vi "WritingAttributes.vi"(0 "reference in":refnum<class "MyG#SubClass.lvclass">, 2 "increment":dbl, 5 "error in (no error)":errorcluster) -> (14 "reference out":refnum<class "MyG#SubClass.lvclass">, 19 "error out":errorcluster)   [LabVIEW 2020, in "MyG#SubClass.lvclass"]
uses:
  MyG#SubClass.lvclass
  C:/Program Files (x86)/National Instruments/LabVIEW 2020/examples/AddQ/G#/CreateDestroy/MyG#Class_class/MyG#Class.lvclass
  MyG#Class_class/MyG#Class.lvclass
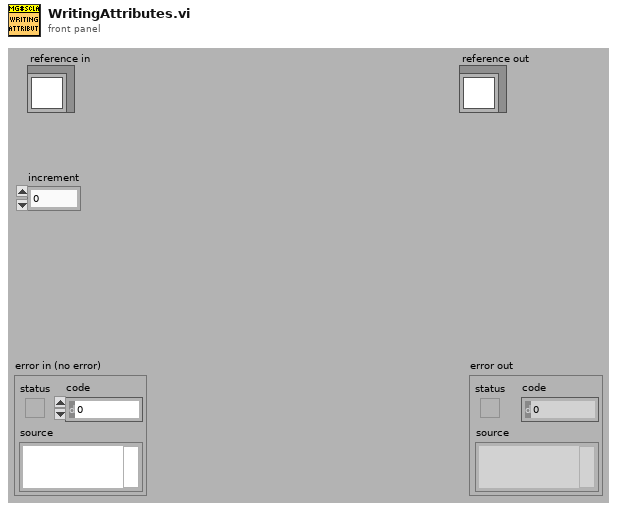
[diagram p1: front panel]
types:
  T1 = typedef "MyG#Class.lvclass/ObjectAttributesRef.ctl" = refnum<data-value>
  T2 = typedef "MyG#SubClass.lvclass/ObjectAttributesRef.ctl" = refnum<data-value>
  T3 = typedef "MyG#SubClass.lvclass/ObjectAttributes.ctl" = cluster{"MySubAttribute":dbl}
  T4 = typedef "MyG#Class.lvclass/ObjectAttributes.ctl" = cluster{"MyAttribute":dbl}
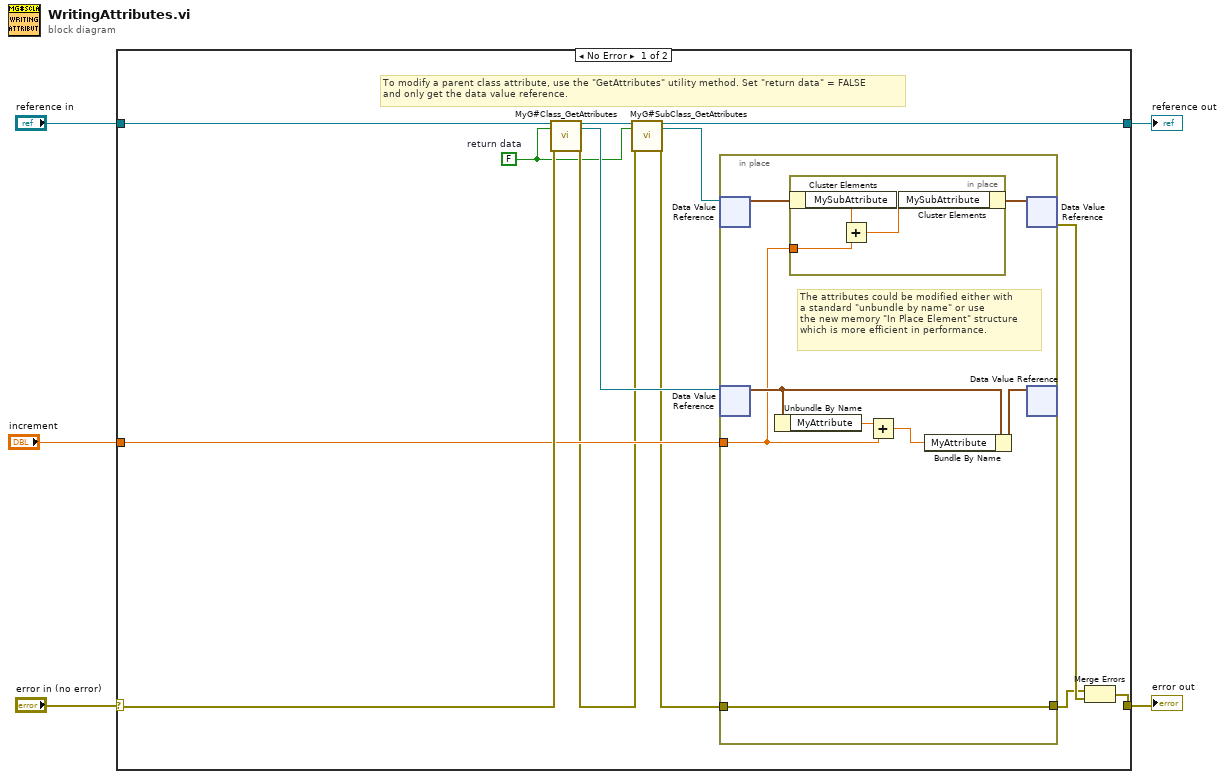
[diagram p0: block diagram]
diagram:
  n1 = case shown="No Error" "error in (no error)" {
    selector: "error in (no error)" -> [w14 w31]
    tunnel: [w18 w31] -> w4
    tunnel: [w8 w30] -> w2
    tunnel: "reference in" -> [w15 w30]
    tunnel: "increment" -> [w12 _]
    frame No Error {
      w7 = FALSE  # return data
      # "To modify a parent class attribute, use the \"GetAttributes\" utility method. Set \"return data\" = FALSE\nand only get the data value reference."
      n2 = call "MyG#Class_GetAttributes.vi"("reference in"=w15, "return data? (T)"=w7, "error in (no error)"=w14) -> ("reference out"=w11:refnum<class "MyG#SubClass.lvclass">, "attributes ref"=w13:T1, "error out"=w10:errorcluster)  [unwired: 13 in, 1 out]
      n3 = call "MyG#SubClass_GetAttributes.vi"("reference in"=w11, "return data? (T)"=w7, "error in (no error)"=w10) -> ("reference out"=w8:refnum<class "MyG#SubClass.lvclass">, "attributes ref"=w6:T2, "error out"=w9:errorcluster)  [unwired: 13 in, 1 out]
      n4 = in-place {
        in-place-border: w9 -> [w24]
        in-place-border: [w24] -> w16
        in-place-border: w12 -> [w19]
        # "The attributes could be modified either with\na standard \"unbundle by name\" or use\nthe new memory \"In Place Element\" structure\nwhich is more efficient in performance."
        n5 = in-place-dvr #1(w6) -> (w25:T3)  [unwired: 1 out]
        n6 = in-place-dvr #2(w13) -> (w22:T4)  [unwired: 1 out]
        n7 = Unbundle By Name(w22) -> ("MyAttribute"=w21:dbl)
        n8 = in-place {
          in-place-border: w19 -> [w28]
          n9 = in-place-cluster #3(w25) -> ("MySubAttribute"=w29:dbl)
          n10 = Add(x=w29, y=w28) -> (x+y=w27:dbl)
          n11 = in-place-cluster #3("MySubAttribute"=w27) -> (w26:T3)
        }
        n12 = Add(x=w21, y=w19) -> (x+y=w20:dbl)
        n13 = Bundle By Name(cluster=w22, "MyAttribute"=w20) -> (w23:T4)
        n14 = in-place-dvr #1(w26) -> (w17:errorcluster)  [unwired: 1 out]
        n15 = in-place-dvr #2(w23) -> ()  [unwired: 2 out]
      }
      n16 = Merge Errors(w16, w17) -> (w18:errorcluster)
    }
    frame Error {
    }
  }
  "error out" <- w4
  "reference out" <- w2
